vi "Revision Query.vi"(8 "error in (no error)":errorcluster {"code" format="%.0x"}, 11 "instrument handle":refnum<k15>) -> (0 "error out":errorcluster {"code" format="%.0x"}, 1 "firmware revision":string, 2 "instrument driver revision":string, 3 "instrument handle out":refnum<k15>)   [LabVIEW 2020, in "Keysight DAQ970.lvlib"]
doc: "Retrieves revision information from the instrument."
uses:
  Keysight DAQ970.lvlib
  KtDAQ970.dll
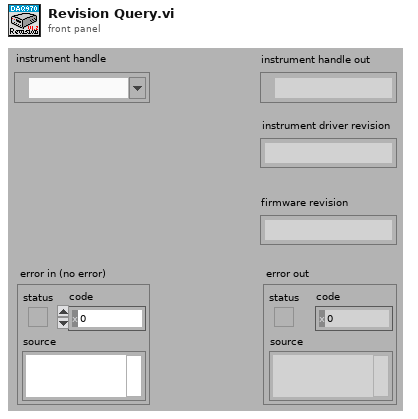
[diagram p1: front panel]
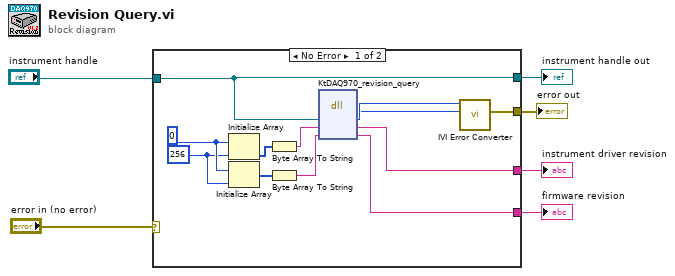
[diagram p0: block diagram]
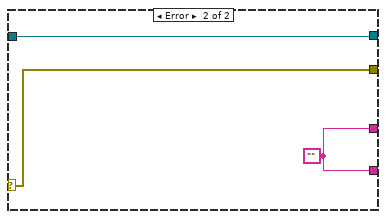
[diagram p2: hidden frame]
diagram:
  n1 = case shown="No Error" "error in (no error)" {
    selector: "error in (no error)" -> [_ w20]
    tunnel: [w13 w20] -> w6
    tunnel: "instrument handle" -> [w7 w21]
    tunnel: [w9 w19] -> w3
    tunnel: [w8 w19] -> w2
    tunnel: [w7 w21] -> w1
    frame No Error {
      w10 = 256
      w11 = u8 0
      n2 = Initialize Array(w11, w10) -> (w18:u8[])
      n3 = Initialize Array(w11, w10) -> (w17:u8[])
      n4 = Byte Array To String(unsigned byte array=w18) -> (string=w16:string)
      n5 = Byte Array To String(unsigned byte array=w17) -> (string=w15:string)
      n6 = dll-call lib="KtDAQ970**.dll" fn="KtDAQ970_revision_query" ("LabVIEW:IviDmm_revision_query")("instrument handle"=w7, "instrument driver revision"=w16, "firmware revision"=w15) -> ("Status"=w12:i32, "instrument handle"=w14:u32, "instrument driver revision"=w9:string, "firmware revision"=w8:string)  [unwired: 3 in, 2 out]
      n7 = call "IVI Error Converter.vi"("IVI error code (0)"=w12, "instrument handle"=w14) -> ("error out"=w13:errorcluster)  [unwired: 8 in, 1 out]
    }
    frame Error {
      w19 = ""
    }
  }
  "error out" <- w6
  "instrument handle out" <- w1
  "instrument driver revision" <- w3
  "firmware revision" <- w2
